vi "Min & Max [[U16]].vi"(2 "Array":u16[][](array[numeric])) -> (5 "Standard Max Indices":i32[](array[numeric]), 6 "Max Value":u16, 7 "Array of Max Indices":T1(array[cluster]), 8 "Standard Min Indices":i32[](array[numeric]), 9 "Min Value":u16, 10 "Array of Min Indices":T1(array[cluster]))   [LabVIEW 2021, in "Arrays.lvlib"]
uses:
  Arrays.lvlib
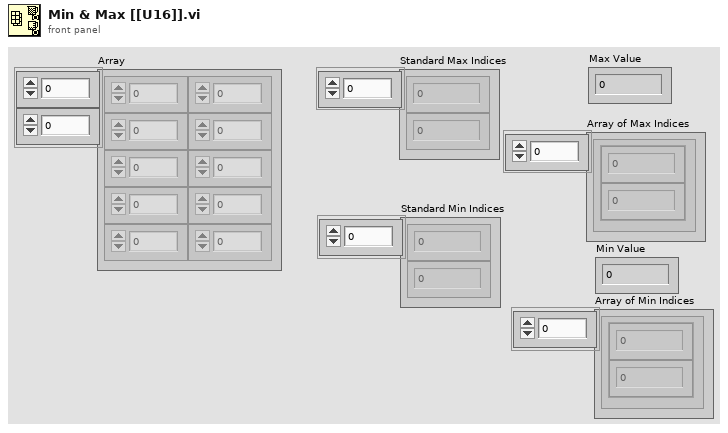
[diagram p1: front panel]
types:
  T1 = cluster{"Numeric Control":i32, "Numeric Control":i32}[]
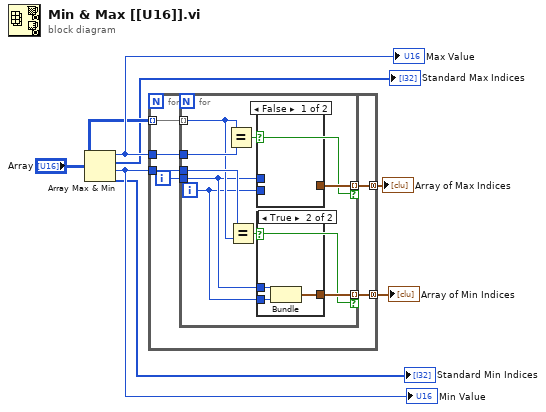
[diagram p0: block diagram]
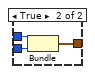
[diagram p3: hidden frame]
diagram:
  n1 = Array Max & Min(array="Array") -> (max value=w7:u16, max index (indices)=→"Standard Max Indices":i32[], min value=w3:u16, min index (indices)=→"Standard Min Indices":i32[])
  "Max Value" <- w7
  "Min Value" <- w3
  n2 = for {
    tunnel: w7 -> [w12]
    tunnel: "Array" -> [w13] mode=indexing
    tunnel: [w10] -> w5 mode=concatenating
    tunnel: w3 -> [w9]
    tunnel: [w8] -> w2 mode=concatenating
    i -> [w11]
    n3 = for {
      tunnel: w13 -> [w18] mode=indexing
      tunnel: w12 -> [w22]
      tunnel: w11 -> [w17]
      tunnel: [w21] -> w10 mode=indexing if=w20
      tunnel: w9 -> [w19]
      tunnel: [w15] -> w8 mode=indexing if=w14
      i -> [w16]
      n4 = Equal?(x=w18, y=w22) -> (x = y?=w20:bool)
      n5 = Equal?(x=w19, y=w18) -> (x = y?=w14:bool)
      n6 = case shown="False" w20 {
        tunnel: w17 -> [_ w28]
        tunnel: w16 -> [_ w27]
        tunnel: [_ w26] -> w21
        frame False {
        }
        frame True {
          n7 = Bundle(w28, w27) -> (w26:cluster{i32, i32})  [unwired: 1 in]
        }
      }
      n8 = case shown="True" w14 {
        tunnel: w17 -> [_ w25]
        tunnel: w16 -> [_ w24]
        tunnel: [_ w23] -> w15
        frame False {
        }
        frame True {
          n9 = Bundle(w25, w24) -> (w23:cluster{i32, i32})  [unwired: 1 in]
        }
      }
    }
  }
  "Array of Max Indices" <- w5
  "Array of Min Indices" <- w2
